vi "Get Value (JSON).vi"(8 "error in (no error)":errorcluster, 10 "key":string, 11 "JSON Object in":refnum<class "JSON Object.lvclass">) -> (0 "error out":errorcluster, 2 "value":refnum<class "JSON Null.lvclass">)   [LabVIEW 2015, in "LVJSON.lvlib" / "JSON Object.lvclass"]
uses:
  JSON Object.lvclass
  JSON Datatype/JSON Null.lvclass
  JSON Object.lvclass/JSON Object.ctl
  Errors/Errors.ctl
  LVJSON.lvlib
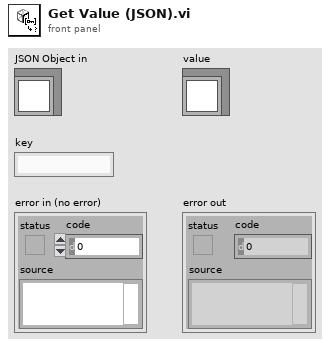
[diagram p1: front panel]
types:
  T1 = typedef "Errors.ctl" = enum16{"No key", "Key path type", "Array OOB", "Type Mismatch"}
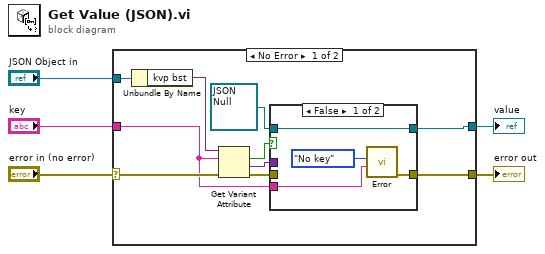
[diagram p0: block diagram]
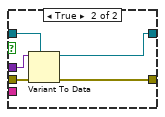
[diagram p2: hidden frame]
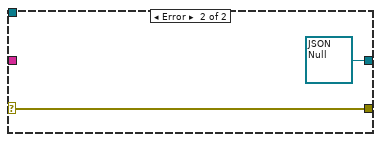
[diagram p3: hidden frame]
diagram:
  n1 = case shown="No Error" "error in (no error)" {
    selector: "error in (no error)" -> [w13 w26]
    tunnel: [w11 w26] -> w4
    tunnel: "JSON Object in" -> [w15 _]
    tunnel: "key" -> [w6 _]
    tunnel: [w9 refnum<class "JSON Null.lvclass"> refnum ("value")] -> w1
    frame No Error {
      n2 = Unbundle By Name(w15) -> ("kvp bst"=w8:variant)
      n3 = Get Variant Attribute(Variant=w8, name=w6, error in=w13) -> (found=w7:bool, value=w14:variant, error out=w12:errorcluster)  [unwired: 1 in, 1 out]
      n4 = case shown="False" w7 {
        tunnel: w14 -> [_ w24]
        tunnel: w12 -> [_ w23]
        tunnel: [w18 w22] -> w11
        tunnel: refnum<class "JSON Null.lvclass"> refnum ("JSON Datatype.lvclass") -> [w19 w21]
        tunnel: [w19 w20] -> w9
        tunnel: w6 -> [w16 _]
        frame False {
          n5 = call "Error.vi"("Data"=w16, "Enum"=Errors."No key") -> ("error out"=w18:errorcluster)  [unwired: 8 in]
        }
        frame True {
          n6 = Variant To Data(error in=w23, type=w21, Variant=w24) -> (data=w20:refnum<class "JSON Null.lvclass">, error out=w22:errorcluster)
        }
      }
    }
    frame Error {
    }
  }
  "error out" <- w4
  "value" <- w1
